vi "DAC Init Results.vi"(8 "error in":errorcluster, 9 "Log Details?":bool, 10 "tdms file":refnum<k34>, 11 "DAC Keller Diff P 23X in":refnum<class "DAC Keller Diff P 23X.lvclass">) -> (0 "error out":errorcluster, 2 "tdms file out":refnum<k34>)   [LabVIEW 2019, in "DAC.lvlib" / "DAC Keller Diff P 23X.lvclass"]
uses:
  DAC Keller Diff P 23X.lvclass
  C:/Users/krio/Documents/LV_Projects/test-stand/App/DAC/DAC.lvclass
  DAC.lvclass/DAC.ctl
  DAC Keller Diff P 23X.lvclass/DAC Keller Diff P 23X.ctl
  DAC.lvclass
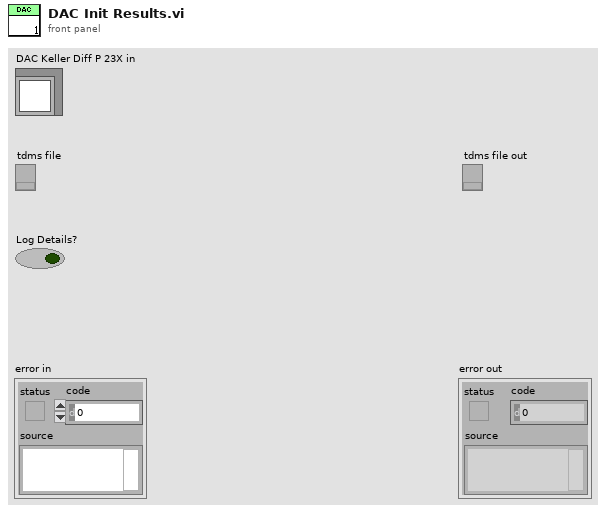
[diagram p1: front panel]
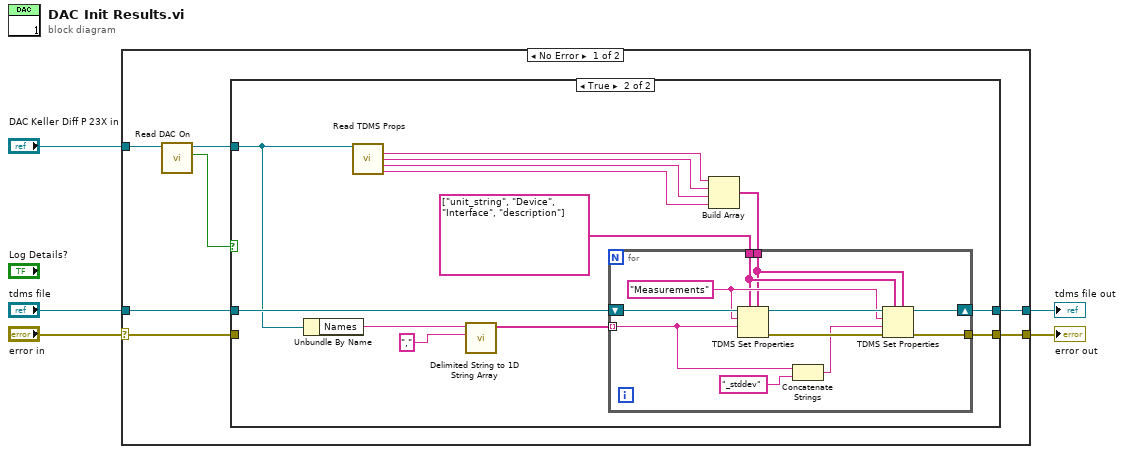
[diagram p0: block diagram]
diagram:
  n1 = case shown="No Error" "error in" {
    selector: "error in" -> [w7 w40]
    tunnel: [w10 w40] -> w2
    tunnel: "DAC Keller Diff P 23X in" -> [w9 _]
    tunnel: "tdms file" -> [w12 w39]
    tunnel: [w11 w39] -> w1
    frame No Error {
      n2 = call "Read DAC On.vi"("DAC in"=w9) -> ("DAC On"=w6:bool, "DAC out"=w8:refnum<class "DAC Keller Diff P 23X.lvclass">)  [unwired: 8 in, 1 out]
      n3 = case shown="True" w6 {
        tunnel: w12 -> [w14 w27]
        tunnel: [w14 w26] -> w11
        tunnel: [w13 w25] -> w10
        tunnel: w8 -> [_ w19]
        tunnel: w7 -> [w13 _]
        frame False {
        }
        frame True {
          n4 = Unbundle By Name(w19) -> ("Names"=w22:string)
          n5 = call "Read TDMS Props.vi"("DAC in"=w19) -> ("Result Unit"=w18:string, "DAC Device"=w17:string, "DAC IO"=w16:string, "DAC Description"=w15:string)  [unwired: 10 in, 1 out]
          n6 = call <vilib>:"Delimited String to 1D String Array.vi"("delimiter"=",", "delimited string"=w22) -> ("string array"=w24:string[])  [unwired: 9 in]
          n7 = Build Array(w18, w17, w16, w15) -> (w21:string[])
          n8 = for {
            tunnel: w24 -> [w32] mode=indexing
            tunnel: string[] ["unit_string", "Device", "Interface", "description"] ("property names") -> [w29]
            tunnel: w21 -> [w28]
            tunnel: [w34] -> w25
            shift-right: [w36] -> w26
            shift-left: w27 -> [w38]
            w30 = "Measurements" ("group name in (Untitled)")
            n9 = TDMS Set Properties(5:w28, 7:w29, 9:w32, 10:w30, 11:w38) -> (0:w35:errorcluster, 3:w37:refnum<k34>)  [unwired: 1 in, 2 out]
            n10 = Concatenate Strings(w32, "_stddev" ("string")) -> (w31:string)
            n11 = TDMS Set Properties(5:w28, 7:w29, 8:w35, 9:w31, 10:w30, 11:w37) -> (0:w34:errorcluster, 3:w36:refnum<k34>)  [unwired: 2 out]
          }
        }
      }
    }
    frame Error {
    }
  }
  "error out" <- w2
  "tdms file out" <- w1
